vi "rcpacini_move_constant_label.vi"(8 "error in (no error)":errorcluster, 11 "Constant in":refnum<vi>) -> (0 "error out":errorcluster, 3 "Constant out":refnum<vi>)   [LabVIEW 2019]
doc: "Move a constant label to the left middle.\n\nCreated by: Ryan Pacini"
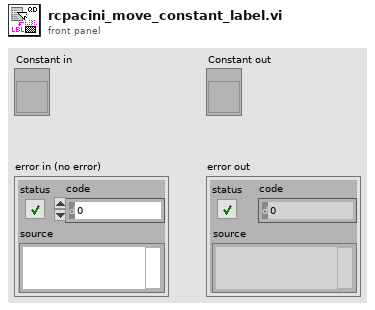
[diagram p1: front panel]
types:
  T1 = typedef "LVRectTypeDef.ctl" = cluster{"Left":i16, "Top":i16, "Right":i16, "Bottom":i16}
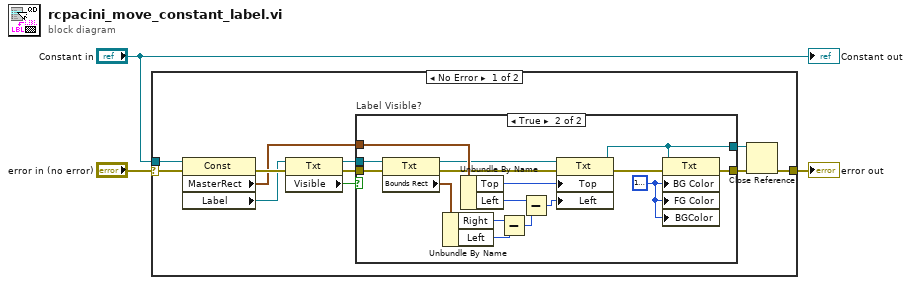
[diagram p0: block diagram]
diagram:
  n1 = case shown="No Error" "error in (no error)" {
    selector: "error in (no error)" -> [w8 w33]
    tunnel: [w9 w33] -> w2
    tunnel: "Constant in" -> [w6 _]
    frame No Error {
      n2 = property class="Const"(reference=w6, error in=w8) -> (error out=w7:errorcluster, "MasterRect"=w4:T1, "Label"=w5:refnum<vi>)  [unwired: 1 out]
      n3 = property class="Txt"(reference=w5, error in=w7) -> (reference out=w12:refnum<vi>, error out=w10:errorcluster, "Visible"=w11:bool)
      n4 = case "Label Visible?" shown="True" w11 {
        tunnel: w10 -> [w16 w32]
        tunnel: w12 -> [w15 w31]
        tunnel: [w16 w28] -> w13
        tunnel: w4 -> [_ w29]
        tunnel: [w15 w27] -> w14
        frame False {
        }
        frame True {
          w26 = u32 16777216
          n5 = property class="Txt"(reference=w31, error in=w32) -> (reference out=w20:refnum<vi>, error out=w21:errorcluster, "Bounds Rect"=w18:T1)
          n6 = Unbundle By Name(w18) -> ("Right"=w24:i16, "Left"=w25:i16)
          n7 = Unbundle By Name(w29) -> ("Top"=w19:i16, "Left"=w22:i16)
          n8 = Subtract(x=w24, y=w25) -> (x-y=w23:i16)
          n9 = Subtract(x=w22, y=w23) -> (x-y=w17:i16)
          n10 = property class="Txt"(reference=w20, error in=w21, "Top"=w19, "Left"=w17) -> (reference out=w27:refnum<vi>, error out=w30:errorcluster)
          n11 = property class="Txt"(reference=w27, error in=w30, "BG Color"=w26, "FG Color"=w26, "BGColor"=w26) -> (error out=w28:errorcluster)  [unwired: 1 out]
        }
      }
      n12 = Close Reference(reference=w14, error in (no error)=w13) -> (error out=w9:errorcluster)
    }
    frame Error {
    }
  }
  "error out" <- w2
  "Constant out" <- "Constant in"
